vi "map_key_polygons.vi"(8 "error in (no error)":errorcluster, 11 "midi-ui in":refnum<class "midi-ui.lvclass">) -> (0 "error out":errorcluster, 3 "midi-ui out":refnum<class "midi-ui.lvclass">)   [LabVIEW 2020, in "midi-ui.lvclass"]
uses:
  midi-ui.lvclass
  midi-ui.lvclass/midi-ui.ctl
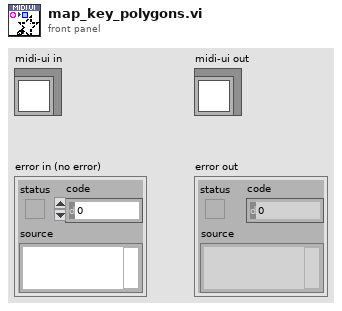
[diagram p1: front panel]
types:
  T1 = typedef "midi-ui.lvclass/privatedata.ctl" = cluster{"White Key Length":dbl, "White Key Width":dbl, "Black Key Length":dbl, "Key Polygon Corners by Name":map{string, cluster{"x":dbl, "y":dbl}[]}, "Anticlockwise rotations [0-3] (0)":i32, "Polygon Corners by Note Name":map{string, cluster{"x":dbl, "y":dbl}[]}, "Picture Control":refnum<vi>, "Owning VI":refnum<vi>, "Control Index":i32, "Note Bounds by Note Name":map{string, cluster{"max":dbl, "min":dbl}}, "Notes on screen":cluster{"Note Value":enum8{"C-2", "C#-2", "D-2", "D#-2", "E-2", "F-2", "F#-2", "G-2", "G#-2", "A-2", "A#-2", "B-2", "C-1", "C#-1", "D-1", "D#-1", "E-1", "F-1", "F#-1", "G-1", "G#-1", "A-1", "A#-1", "B-1", "C0", "C#0", "D0", "D#0", "E0", "F0", "F#0", "G0", "G#0", "A0", "A#0", "B0", "C1", "C#1", "D1", "D#1", "E1", "F1", "F#1", "G1", "G#1", "A1", "A#1", "B1", "C2", "C#2", "D2", "D#2", "E2", "F2", "F#2", "G2", "G#2", "A2", "A#2", "B2", "C3", "C#3", "D3", "D#3", "E3", "F3", "F#3", "G3", "G#3", "A3", "A#3", "B3", "C4", "C#4", "D4", "D#4", "E4", "F4", "F#4", "G4", "G#4", "A4", "A#4", "B4", "C5", "C#5", "D5", "D#5", "E5", "F5", "F#5", "G5", "G#5", "A5", "A#5", "B5", "C6", "C#6", "D6", "D#6", "E6", "F6", "F#6", "G6", "G#6", "A6", "A#6", "B6", "C7", "C#7", "D7", "D#7", "E7", "F7", "F#7", "G7", "G#7", "A7", "A#7", "B7", "C8", "C#8", "D8", "D#8", "E8", "F8", "F#8", "G"}, "End Time":u32, "Start Time":u32}[], "Polygon Pictures by Note Name":map{i32, cluster{"Note On":picture, "Note Off":picture}}, "keyboard":picture[], "Keyboard Note Index by Name":map{i32, i32}, "music":picture[]}
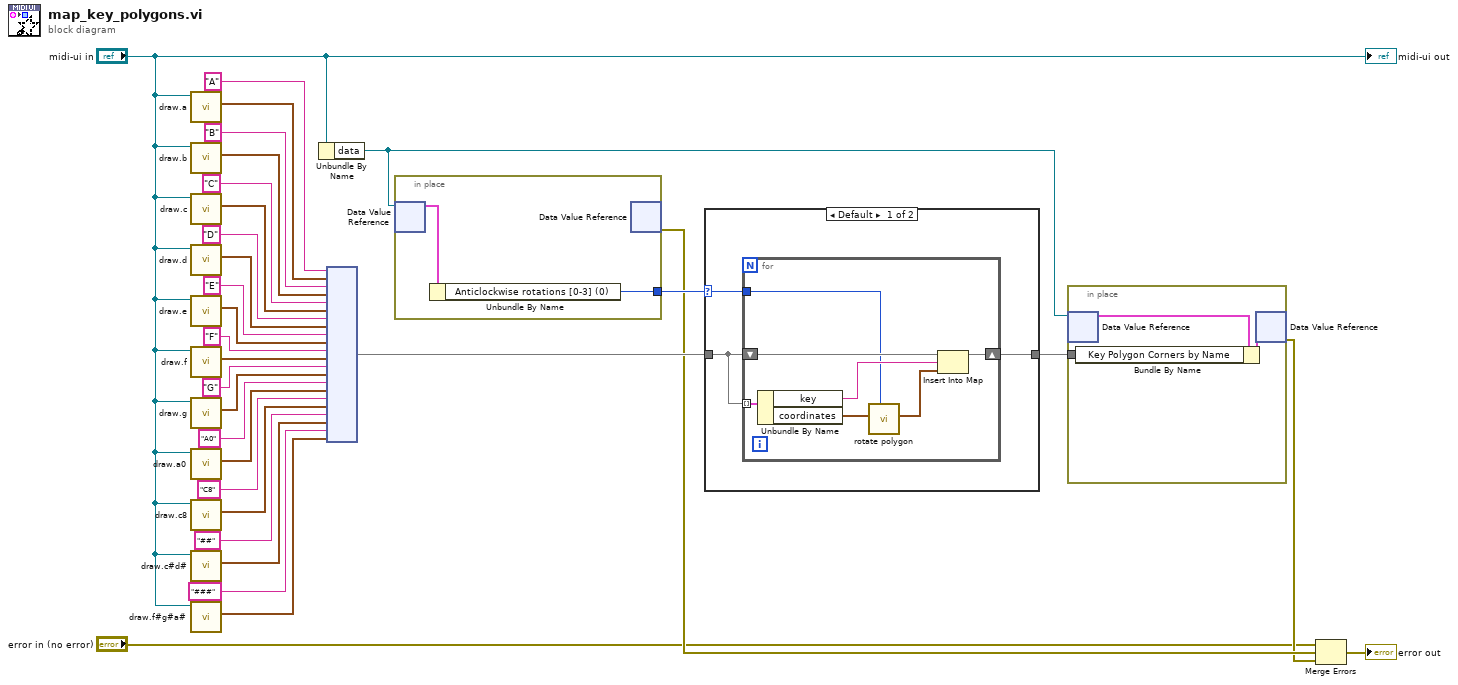
[diagram p0: block diagram]
diagram:
  n1 = call "draw.a.vi"("midi-ui in"="midi-ui in") -> ("coordinates"=w18:cluster{"x":dbl, "y":dbl}[])  [unwired: 9 in, 1 out]
  n2 = call "draw.b.vi"("midi-ui in"="midi-ui in") -> ("coordinates"=w19:cluster{"x":dbl, "y":dbl}[])  [unwired: 9 in, 1 out]
  n3 = call "draw.c.vi"("midi-ui in"="midi-ui in") -> ("coordinates"=w20:cluster{"x":dbl, "y":dbl}[])  [unwired: 9 in, 1 out]
  n4 = call "draw.d.vi"("midi-ui in"="midi-ui in") -> ("coordinates"=w21:cluster{"x":dbl, "y":dbl}[])  [unwired: 9 in, 1 out]
  n5 = call "draw.e.vi"("midi-ui in"="midi-ui in") -> ("coordinates"=w22:cluster{"x":dbl, "y":dbl}[])  [unwired: 9 in, 1 out]
  n6 = call "draw.f.vi"("midi-ui in"="midi-ui in") -> ("coordinates"=w23:cluster{"x":dbl, "y":dbl}[])  [unwired: 9 in, 1 out]
  n7 = call "draw.g.vi"("midi-ui in"="midi-ui in") -> ("coordinates"=w24:cluster{"x":dbl, "y":dbl}[])  [unwired: 9 in, 1 out]
  n8 = call "draw.a0.vi"("midi-ui in"="midi-ui in") -> ("coordinates"=w14:cluster{"x":dbl, "y":dbl}[])  [unwired: 9 in, 1 out]
  n9 = call "draw.c8.vi"("midi-ui in"="midi-ui in") -> ("coordinates"=w15:cluster{"x":dbl, "y":dbl}[])  [unwired: 9 in, 1 out]
  n10 = call "draw.c#d#.vi"("midi-ui in"="midi-ui in") -> ("coordinates"=w12:cluster{"x":dbl, "y":dbl}[])  [unwired: 9 in, 1 out]
  n11 = call "draw.f#g#a#.vi"("midi-ui in"="midi-ui in") -> ("coordinates"=w13:cluster{"x":dbl, "y":dbl}[])  [unwired: 9 in, 1 out]
  n12 = Unbundle By Name("midi-ui in") -> ("data"=w6:refnum<data-value>)
  n13 = node("A" ("key"), w18, "B" ("key"), w19, "C" ("key"), w20, "D" ("key"), w21, "E" ("key"), w22, "F" ("key"), w23, "G" ("key"), w24, "A0" ("key"), w14, "C8" ("key"), w15, "##" ("key"), w12, "###" ("key"), w13) -> (w9:map{string, cluster{"x":dbl, "y":dbl}[]})
  n14 = in-place {
    in-place-border: [w32] -> w5
    n15 = in-place-dvr #1(w6) -> (w33:T1)  [unwired: 1 out]
    n16 = Unbundle By Name(w33) -> ("Anticlockwise rotations [0-3] (0)"=w32:i32)
    n17 = in-place-dvr #1() -> (w4:errorcluster)  [unwired: 1 in, 1 out]
  }
  n18 = case shown="Default" w5 {
    selector: w5 -> [w34 _]
    tunnel: w9 -> [w36 w44]
    tunnel: [w35 w44] -> w8
    frame Default {
      n19 = for {
        tunnel: w36 -> [w43] mode=indexing
        shift-right: [w41] -> w35
        shift-left: w36 -> [w42]
        tunnel: w34 -> [w37]
        n20 = Unbundle By Name(w43) -> ("key"=w40:string, "coordinates"=w39:cluster{"x":dbl, "y":dbl}[])
        n21 = call "rotate polygon.vi"("Anticlockwise rotations [0-3] (0)"=w37, "Polygon Corners in"=w39) -> ("Rotated Polygone Corners out"=w38:cluster{"x":dbl, "y":dbl}[])  [unwired: 9 in]
        n22 = Insert Into Map(map in=w42, key=w40, value=w38) -> (map out=w41:map{string, cluster{"x":dbl, "y":dbl}[]})  [unwired: 2 out]
      }
    }
    frame 0 {
    }
  }
  n23 = in-place {
    in-place-border: w8 -> [w46]
    n24 = in-place-dvr #2(w6) -> (w47:T1)  [unwired: 1 out]
    n25 = Bundle By Name(cluster=w47, "Key Polygon Corners by Name"=w46) -> (w45:T1)
    n26 = in-place-dvr #2(w45) -> (w3:errorcluster)  [unwired: 1 out]
  }
  n27 = Merge Errors("error in (no error)", w4, w3) -> (→"error out":errorcluster)
  "midi-ui out" <- "midi-ui in"
